vi "Message Enqueue.vi"(6 "Priority?":bool, 8 "error in (no error)":errorcluster, 9 "Value":variant, 10 "Message":string, 11 "Message Queue":refnum<queue>) -> (0 "error out":errorcluster, 3 "Message Queue dup":refnum<queue>)   [LabVIEW 2013]
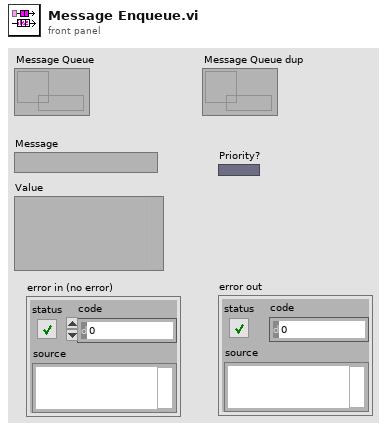
[diagram p1: front panel]
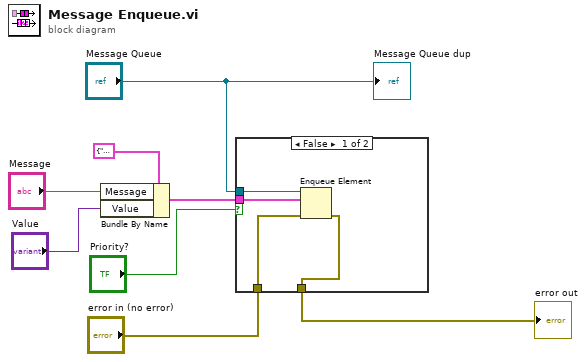
[diagram p0: block diagram]
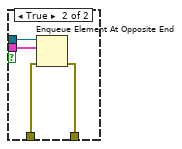
[diagram p2: hidden frame]
diagram:
  n1 = Bundle By Name(cluster=cluster{"Message":string, "Value":variant} {"Message"="", "Value"=variant} ("Message Cluster"), "Message"="Message", "Value"="Value") -> (w6:cluster{"Message":string, "Value":variant})
  n2 = case shown="False" "Priority?" {
    tunnel: "Message Queue" -> [w12 w16]
    tunnel: w6 -> [w11 w15]
    tunnel: "error in (no error)" -> [w10 w14]
    tunnel: [w9 w13] -> w3
    frame False {
      n3 = Enqueue Element(queue=w12, element=w11, error in (no error)=w10) -> (error out=w9:errorcluster)  [unwired: 1 in, 2 out]
    }
    frame True {
      n4 = Enqueue Element At Opposite End(queue=w16, element=w15, error in (no error)=w14) -> (error out=w13:errorcluster)  [unwired: 1 in, 2 out]
    }
  }
  "error out" <- w3
  "Message Queue dup" <- "Message Queue"
